vi "Translate Arduino Data.vi"(0 "Analog Port In":dbl[](array[numeric]), 1 "Median Filter Rank":i32=2) -> (2 "Front Left (Pin 0)":cluster{u32, u32}(slide) scale=0.0..1000.0, 3 "Sonar Data":cluster{dbl, dbl, dbl}, 4 "Front Center (Pin 1)":cluster{u32, u32}(slide) scale=0.0..1000.0, 5 "Front Right (Pin 2)":cluster{u32, u32}(slide) scale=0.0..1000.0, 6 "Rear Left (Pin 3)":cluster{dbl, dbl}(slide) scale=1.0..1000.0 scale format="%#_4g", 7 "Rear Right (Pin 4)":cluster{dbl, dbl}(slide) scale=1.0..1000.0 scale format="%#_4g")   [LabVIEW 2011]
uses:
  <vilib>/ptbypt/NI_PtbyPt.lvlib
panel:
  out "Pin 5":dbl
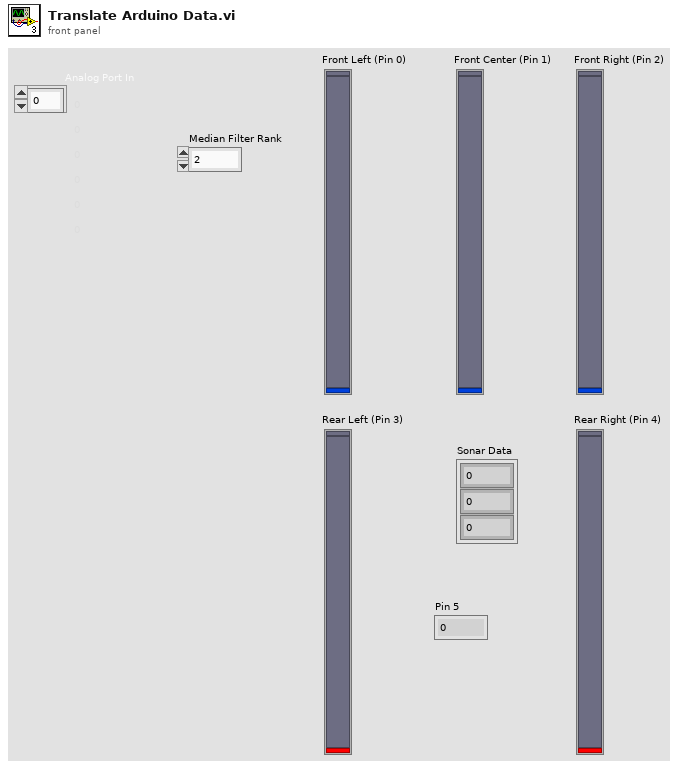
[diagram p1: front panel]
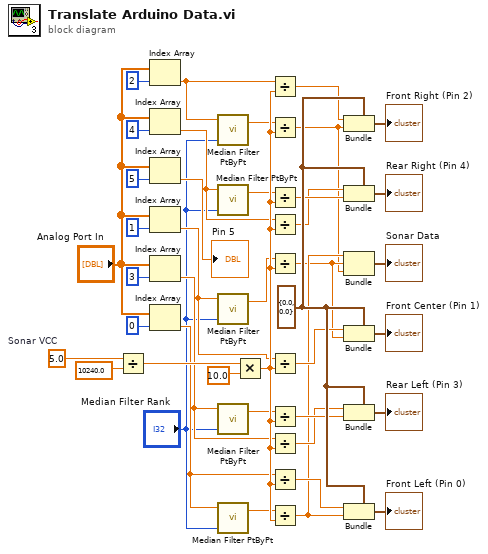
[diagram p0: block diagram]
diagram:
  w25 = cluster{dbl, dbl} {0.0, 0.0} ("Front Left (Pin 0) 2")
  w35 = 5.0  # Sonar VCC
  n1 = Divide(x=w35, y=10240.0) -> (x/y=w33:dbl)
  n2 = Index Array(array="Analog Port In", index=2) -> (element=w21:dbl)
  n3 = Index Array(array="Analog Port In", index=4) -> (element=w20:dbl)
  n4 = Index Array(array="Analog Port In", index=5) -> (element=→"Pin 5":dbl)
  n5 = Index Array(array="Analog Port In", index=1) -> (element=w17:dbl)
  n6 = Index Array(array="Analog Port In", index=3) -> (element=w13:dbl)
  n7 = Index Array(array="Analog Port In", index=0) -> (element=w15:dbl)
  n8 = call <vilib>:"Median Filter PtByPt.vi"("rank"="Median Filter Rank", "x"=w21) -> ("Filtered x"=w22:dbl)  [unwired: 2 in, 1 out]
  n9 = call <vilib>:"Median Filter PtByPt.vi"("rank"="Median Filter Rank", "x"=w20) -> ("Filtered x"=w19:dbl)  [unwired: 2 in, 1 out]
  n10 = call <vilib>:"Median Filter PtByPt.vi"("rank"="Median Filter Rank", "x"=w17) -> ("Filtered x"=w16:dbl)  [unwired: 2 in, 1 out]
  n11 = call <vilib>:"Median Filter PtByPt.vi"("rank"="Median Filter Rank", "x"=w13) -> ("Filtered x"=w18:dbl)  [unwired: 2 in, 1 out]
  n12 = call <vilib>:"Median Filter PtByPt.vi"("rank"="Median Filter Rank", "x"=w15) -> ("Filtered x"=w14:dbl)  [unwired: 2 in, 1 out]
  n13 = Multiply(x=w33, y=10.0) -> (x*y=w24:dbl)
  n14 = Divide(x=w21, y=w24) -> (x/y=w11:dbl)
  n15 = Divide(x=w22, y=w24) -> (x/y=w2:dbl)
  n16 = Divide(x=w19, y=w24) -> (x/y=w10:dbl)
  n17 = Divide(x=w20, y=w24) -> (x/y=w9:dbl)
  n18 = Divide(x=w16, y=w24) -> (x/y=w3:dbl)
  n19 = Divide(x=w17, y=w24) -> (x/y=w8:dbl)
  n20 = Divide(x=w18, y=w24) -> (x/y=w7:dbl)
  n21 = Divide(x=w13, y=w24) -> (x/y=w6:dbl)
  n22 = Divide(x=w15, y=w24) -> (x/y=w5:dbl)
  n23 = Divide(x=w14, y=w24) -> (x/y=w4:dbl)
  n24 = Bundle(cluster=w25, w11, w2) -> (→"Front Right (Pin 2)":cluster{dbl, dbl})
  n25 = Bundle(cluster=w25, w9, w10) -> (→"Rear Right (Pin 4)":cluster{dbl, dbl})
  n26 = Bundle(w4, w3, w2) -> (→"Sonar Data":cluster{dbl, dbl, dbl})  [unwired: 1 in]
  n27 = Bundle(cluster=w25, w8, w3) -> (→"Front Center (Pin 1)":cluster{dbl, dbl})
  n28 = Bundle(cluster=w25, w6, w7) -> (→"Rear Left (Pin 3)":cluster{dbl, dbl})
  n29 = Bundle(cluster=w25, w5, w4) -> (→"Front Left (Pin 0)":cluster{dbl, dbl})
